vi "32路模拟量输入.vi"() -> ()   [LabVIEW 2010]
uses:
  全局量/全局_配置.vi
panel:
  in  "同步_1":i32
  in  "数组_反馈值":dbl[][](array[numeric])
  in  "第几个数据":i32
  in  "第几组数据":i32
  out "数组_AD幅值":sgl[](array[numeric])
  out "数组_DSP幅值":sgl[](array[numeric])
  in  "数组_设定值":dbl[][](array[numeric])
  in  "数组_选择":bool[](array[boolean])
  out "light_32":bool
  out "light_31":bool
  out "light_30":bool
  out "light_29":bool
  out "light_28":bool
  out "light_27":bool
  out "light_26":bool
  out "light_25":bool
  out "light_24":bool
  out "light_23":bool
  out "light_22":bool
  out "light_21":bool
  out "light_20":bool
  out "light_19":bool
  out "light_18":bool
  out "light_17":bool
  out "Analog_back":string[][](table) caption="表格"
  in  "A_32":bool
  in  "A_31":bool
  in  "A_30":bool
  in  "A_29":bool
  in  "A_28":bool
  in  "A_27":bool
  in  "A_26":bool
  in  "A_25":bool
  in  "A_24":bool
  in  "A_23":bool
  in  "A_22":bool
  in  "A_21":bool
  in  "A_20":bool
  in  "A_19":bool
  in  "A_18":bool
  in  "A_17":bool
  out "合格？":bool[][](array[boolean])
  out "测试结论":string
  out "light_16":bool
  out "light_15":bool
  out "light_14":bool
  out "light_13":bool
  out "light_12":bool
  out "light_11":bool
  out "light_10":bool
  out "light_9":bool
  out "light_8":bool
  out "light_7":bool
  out "light_6":bool
  out "light_5":bool
  out "light_4":bool
  out "light_3":bool
  out "light_2":bool
  out "light_1":bool
  out "退出？":bool
  in  "btn_反选":bool
  in  "btn_全选":bool
  in  "A_16":bool
  in  "A_15":bool
  in  "A_14":bool
  in  "A_13":bool
  in  "A_12":bool
  in  "A_11":bool
  in  "A_10":bool
  in  "A_9":bool
  in  "A_8":bool
  in  "A_7":bool
  in  "A_6":bool
  in  "A_5":bool
  in  "A_4":bool
  in  "A_3":bool
  in  "A_2":bool
  in  "A_1":bool
  in  "btn_取消":bool
  in  "btn_开始测试":bool
  in  "Analog_IN":string[][](table) caption="表格"
  out "Analog_WC":string[][](table) caption="表格"
  # "模拟量选择及输入值（V）"
  # "模拟量反馈值（V）"
  # "模拟量误差值（%）"
  # "测试结论："
  # "从0开始"
  # "从1开始,第0列没有使用"
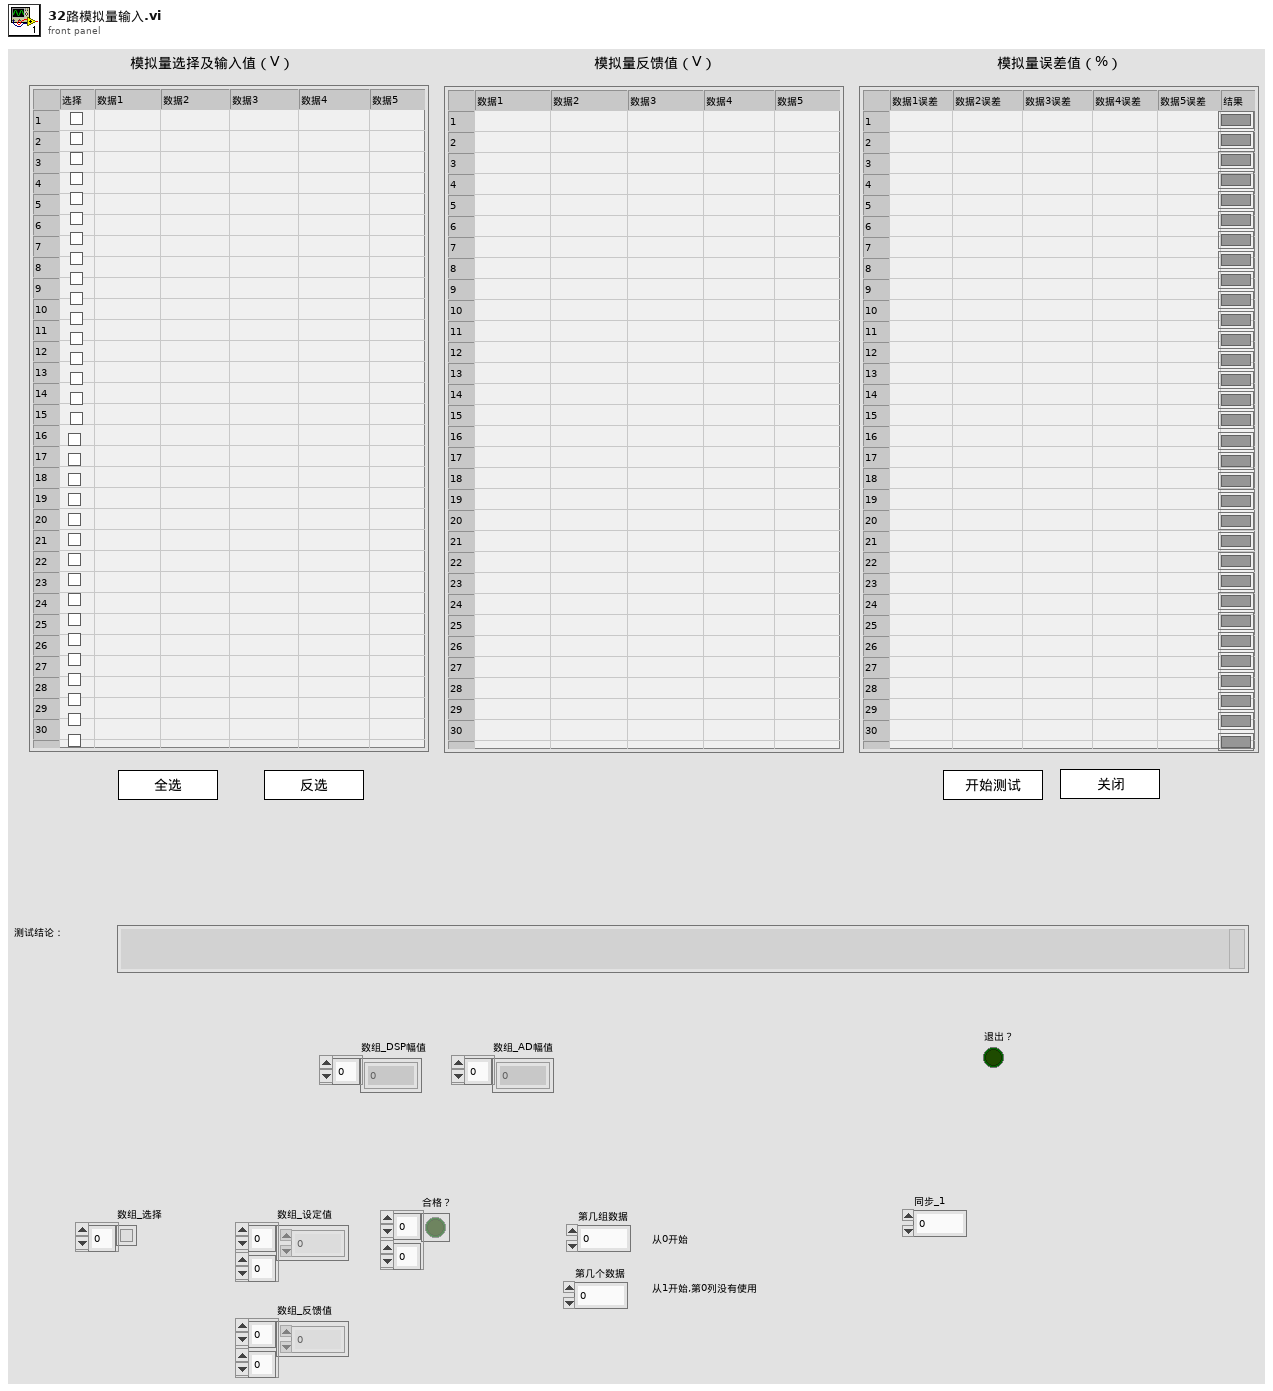
[diagram p1: front panel]
types:
  T1 = enum8{"Enabled", "Disabled", "Disabled and Grayed Out"}
  T2 = cluster{"数字量输入信号路数":u32, "数字量输出信号路数":u32, "DSP模拟量输入信号路数":u32, "DSP模拟量输入信号幅值":u32, "AD模拟量输入信号路数":u32, "AD模拟量输入信号幅值":u32, "RS232端口":u32, "RS232通信路数":u32, "RS232波特率":u32, "RS485端口":u32, "RS485通信路数":u32, "RS485波特率":u32, "CAN通信端口":string, "CAN波特率":u32, "以太网选择?":bool, "控制板IP":string, "以太网端口":u32}
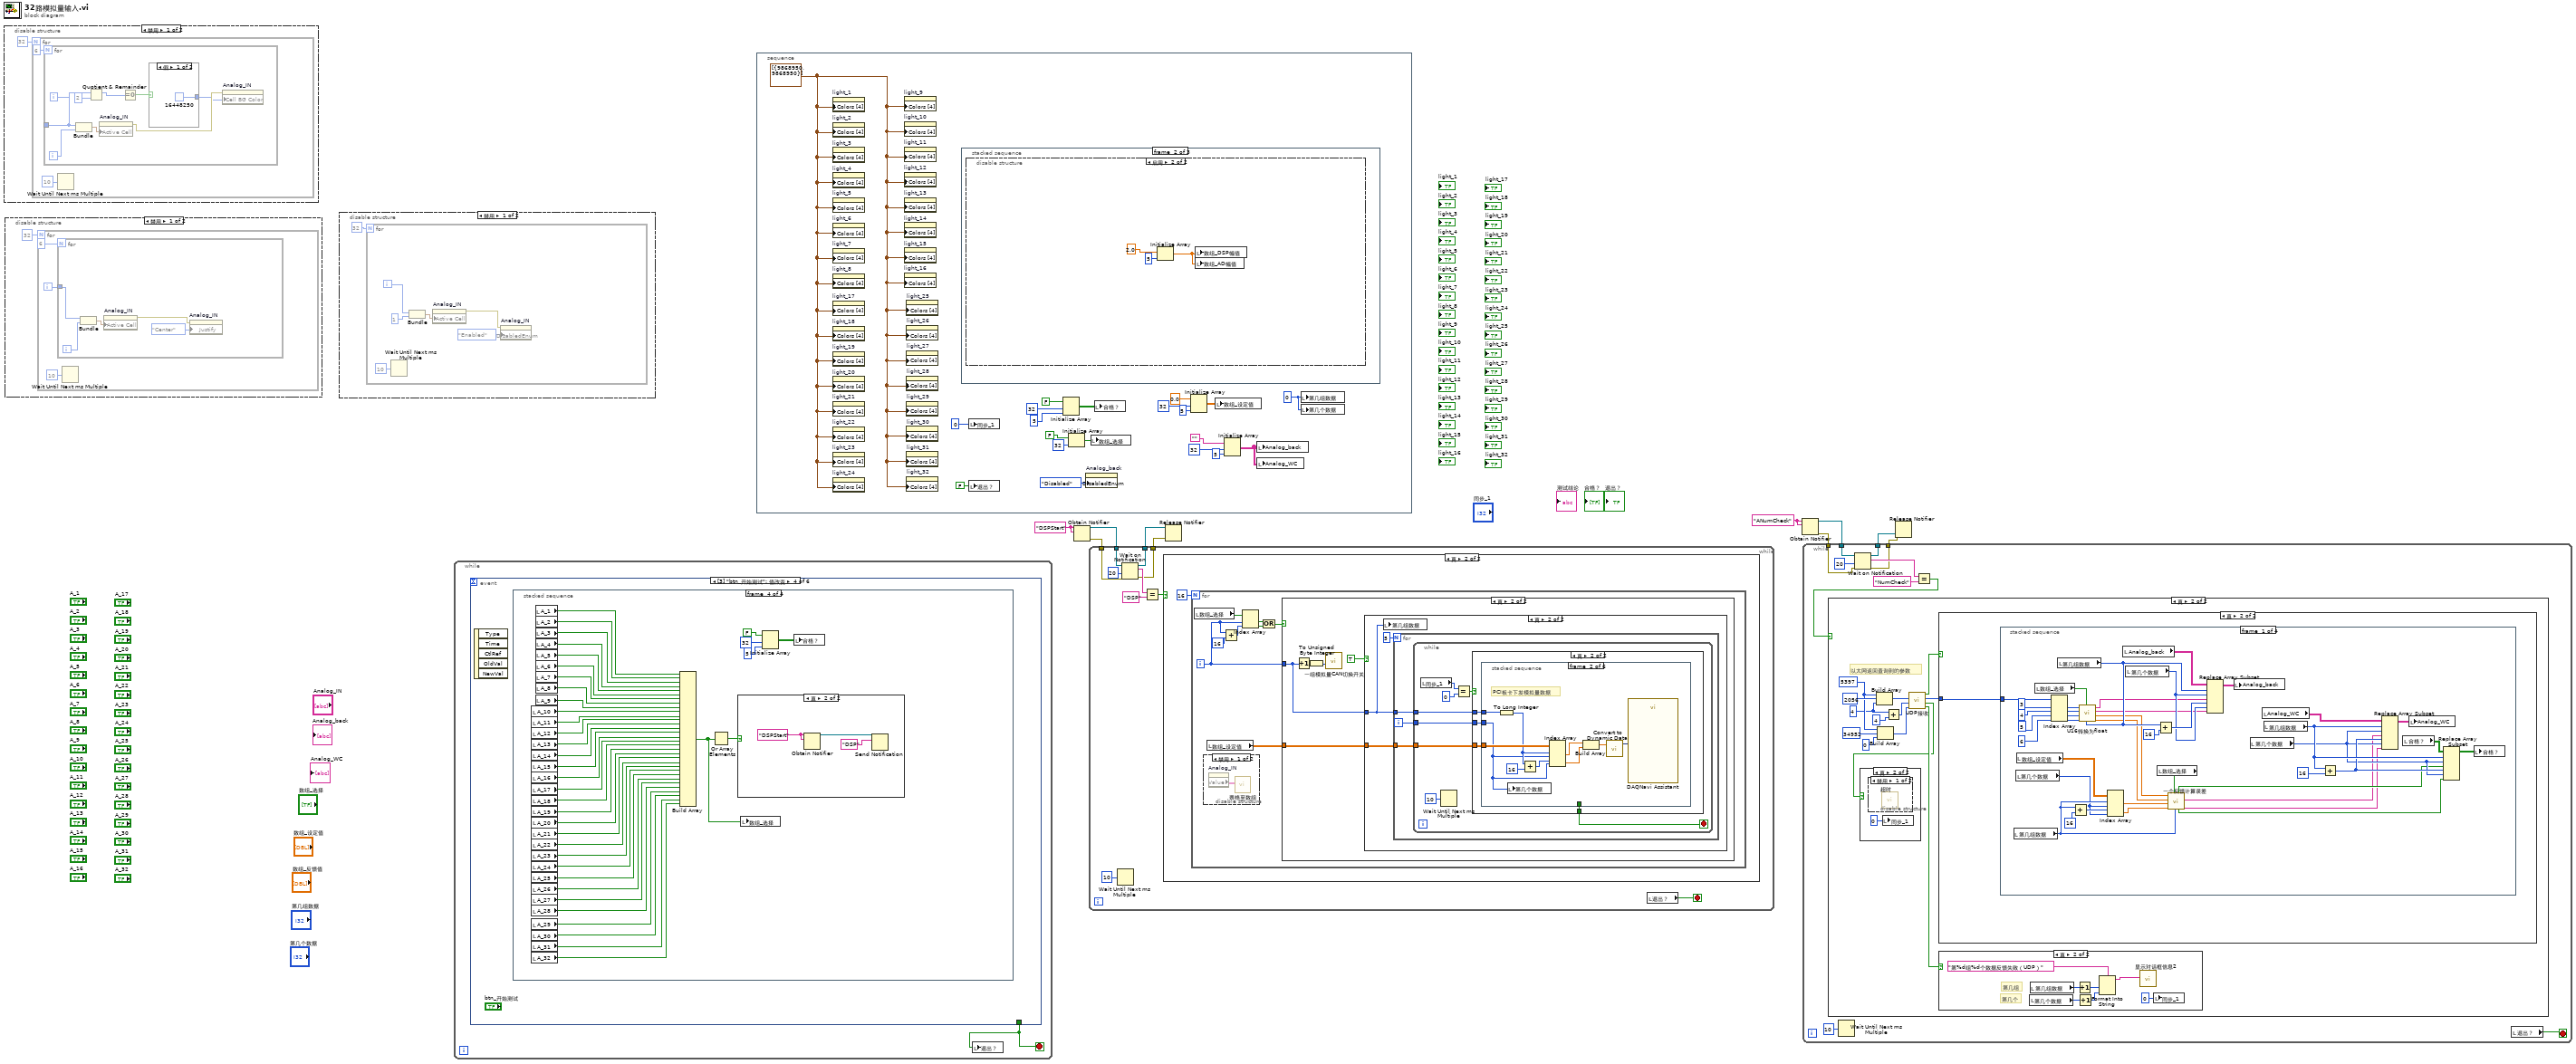
[diagram p0: block diagram]
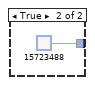
[diagram p2: hidden frame]
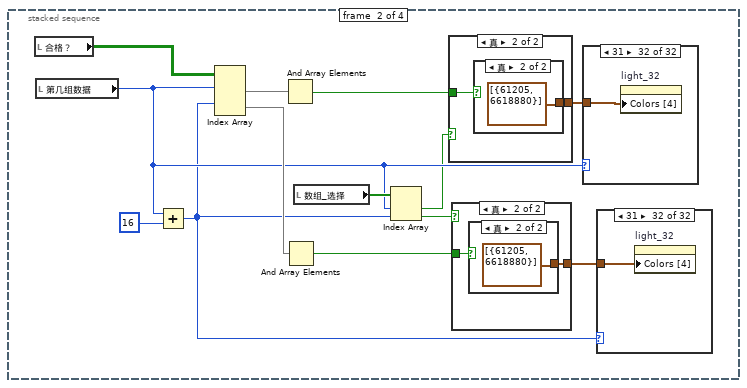
[diagram p9: hidden frame]
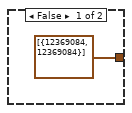
[diagram p10: hidden frame]
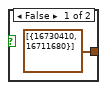
[diagram p11: hidden frame]
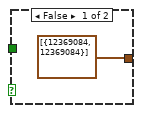
[diagram p12: hidden frame]
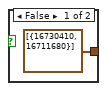
[diagram p13: hidden frame]
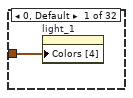
[diagram p14: hidden frame]
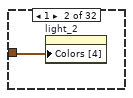
[diagram p15: hidden frame]
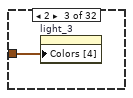
[diagram p16: hidden frame]
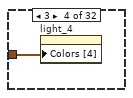
[diagram p17: hidden frame]
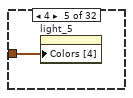
[diagram p18: hidden frame]
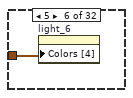
[diagram p19: hidden frame]
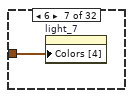
[diagram p20: hidden frame]
diagram:
  w5 = "ANumCheck" ("名称（未命名）")
  w8 = "DSPStart" ("名称（未命名）")
  n1 = disable-structure shown="禁用" {
    frame Disabled {
      n2 = for {
        N: 32 -> [_]
        i -> [w13]
        n3 = for {
          N: 6 -> [_]
          tunnel: w13 -> [w21]
          i -> [w15]
          n4 = Bundle(w21, w15) -> (w18:cluster{i32, i32})  [unwired: 1 in]
          n5 = Quotient & Remainder(x=w21, y=2) -> (x-y*floor(x/y)=w19:i32)  [unwired: 1 out]
          n6 = property on="Analog_IN" class="Tbl (严格)"("Active Cell"=w18) -> (error out=w17:errorcluster)  [unwired: 2 in, 1 out]
          n7 = Equal To 0?(x=w19) -> (x = 0?=w22:bool)
          n8 = case shown="假" w22 {
            tunnel: [u32 16448250 u32 15723488] -> w16
            frame False {
            }
            frame True {
            }
          }
          n9 = property on="Analog_IN" class="Tbl (严格)"(error in=w17, "Cell BG Color"=w16) -> ()  [unwired: 1 in, 2 out]
        }
        n10 = Wait Until Next ms Multiple(millisecond multiple=u32 10 ("毫秒倍数")) -> ()  [unwired: 1 out]
      }
    }
    frame Enabled {
    }
  }
  n11 = disable-structure shown="禁用" {
    frame Disabled {
      n12 = for {
        N: 32 -> [_]
        i -> [w26]
        n13 = for {
          N: 6 -> [_]
          tunnel: w26 -> [w29]
          i -> [w30]
          n14 = Bundle(w29, w30) -> (w33:cluster{i32, i32})  [unwired: 1 in]
          n15 = property on="Analog_IN" class="Tbl (严格)"("Active Cell"=w33) -> (error out=w31:errorcluster)  [unwired: 2 in, 1 out]
          n16 = property on="Analog_IN" class="Tbl (严格)"(error in=w31, "Justify"=enum16{"Left", "Center", "Right"}."Center" ("活动单元格:单元格对齐")) -> ()  [unwired: 1 in, 2 out]
        }
        n17 = Wait Until Next ms Multiple(millisecond multiple=u32 10 ("毫秒倍数")) -> ()  [unwired: 1 out]
      }
    }
    frame Enabled {
    }
  }
  n18 = disable-structure shown="禁用" {
    frame Disabled {
      n19 = for {
        N: 32 -> [_]
        i -> [w39]
        n20 = Wait Until Next ms Multiple(millisecond multiple=u32 10 ("毫秒倍数")) -> ()  [unwired: 1 out]
        n21 = Bundle(w39, 1) -> (w38:cluster{i32, i32})  [unwired: 1 in]
        n22 = property on="Analog_IN" class="Tbl (严格)"("Active Cell"=w38) -> (error out=w35:errorcluster)  [unwired: 2 in, 1 out]
        n23 = property on="Analog_IN" class="Tbl (严格)"(error in=w35, "DisabledEnum"=T1."Enabled" ("禁用")) -> ()  [unwired: 1 in, 2 out]
      }
    }
    frame Enabled {
    }
  }
  n24 = while {
    stop <- w41 stop-if-true
    n25 = event shown="[3] \"btn_开始测试\": 值改变" {
      selector: _ -> [_ _ _ _ _ _]
      dyn-events: _ -> [_ _ _ _ _ _]
      timeout: _ -> [_ _ _ _ _ _]
      tunnel: [_ TRUE TRUE _ _ _] -> w41
      event Timeout {
        n26 = event-data() -> ()  [unwired: 1 in, 2 out]
      }
      event Panel Close {
        n27 = event-data() -> ()  [unwired: 1 in, 3 out]
      }
      event "btn_取消": Value Change {
        n28 = event-data() -> ()  [unwired: 1 in, 5 out]
      }
      event "btn_开始测试": Value Change {
        n29 = event-data() -> ()  [unwired: 1 in, 5 out]
        n30 = stacked-sequence {
          frame #0 {
            w44 = 0 ("第几组数据")
            n31 = local read "Analog_IN"() -> (w51:string[][])
            n32 = Delete From Array(array=w51, length=1 ("长度"), index (col)=0 ("禁用的索引 (列)")) -> (array with subset deleted=w47:string[][])  [unwired: 1 in, 1 out]
            n33 = for {
              N: 32 -> [_]
              tunnel: w47 -> [w54] mode=indexing
              tunnel: [w53] -> w50 mode=indexing
              n34 = for {
                N: 5 -> [_]
                tunnel: w54 -> [w56] mode=indexing
                tunnel: [w55] -> w53 mode=indexing
                n35 = Fract/Exp String To Number(string=w56) -> (number=w55:dbl)  [unwired: 3 in, 1 out]
              }
            }
            n36 = local write "第几组数据"(w44) -> ()
            n37 = local write "第几个数据"(w44) -> ()
            n38 = local write "同步_1"(0 ("同步_2")) -> ()
            n39 = local write "数组_设定值"(w50) -> ()
          }
          frame #1 {
            n40 = local read "Analog_back"() -> (w59:string[][])
            n41 = local read "Analog_WC"() -> (w58:string[][])
            n42 = for {
              tunnel: w58 -> [w95] mode=indexing
              i -> [w94]
              n43 = for {
                tunnel: w95 -> [_] mode=indexing
                tunnel: w94 -> [w99]
                i -> [w98]
                n44 = local read "Analog_WC"() -> (w100:string[][])
                n45 = Replace Array Subset(array=w100, new element="", index (row)=w99, index (col)=w98) -> (w96:string[][])
                n46 = local write "Analog_WC"(w96) -> ()
              }
            }
            n47 = for {
              tunnel: w59 -> [w102] mode=indexing
              i -> [w101]
              n48 = for {
                tunnel: w102 -> [_] mode=indexing
                tunnel: w101 -> [w106]
                i -> [w105]
                n49 = local read "Analog_back"() -> (w107:string[][])
                n50 = Replace Array Subset(array=w107, new element="", index (row)=w106, index (col)=w105) -> (w103:string[][])
                n51 = local write "Analog_back"(w103) -> ()
              }
            }
            n52 = for {
              N: 32 -> [_]
              i -> [w61]
              n53 = case shown="31" w61 {
                tunnel: cluster{u32, u32}[] [{9868950, 9868950}] -> [w62 w63 w64 w65 w66 w67 w68 w69 w70 w71 w72 w73 w74 w75 w76 w77 w78 w79 w80 w81 w82 w83 w84 w85 w86 w87 w88 w89 w90 w91 w92 w93]
                frame 0, Default {
                  n54 = property on="light_1" class="Bool (严格)"("Colors [4]"=w62) -> ()  [unwired: 2 in, 2 out]
                }
                frame 1 {
                  n55 = property on="light_2" class="Bool (严格)"("Colors [4]"=w63) -> ()  [unwired: 2 in, 2 out]
                }
                frame 2 {
                  n56 = property on="light_3" class="Bool (严格)"("Colors [4]"=w64) -> ()  [unwired: 2 in, 2 out]
                }
                frame 3 {
                  n57 = property on="light_4" class="Bool (严格)"("Colors [4]"=w65) -> ()  [unwired: 2 in, 2 out]
                }
                frame 4 {
                  n58 = property on="light_5" class="Bool (严格)"("Colors [4]"=w66) -> ()  [unwired: 2 in, 2 out]
                }
                frame 5 {
                  n59 = property on="light_6" class="Bool (严格)"("Colors [4]"=w67) -> ()  [unwired: 2 in, 2 out]
                }
                frame 6 {
                  n60 = property on="light_7" class="Bool (严格)"("Colors [4]"=w68) -> ()  [unwired: 2 in, 2 out]
                }
                frame 7 {
                  n61 = property on="light_8" class="Bool (严格)"("Colors [4]"=w69) -> ()  [unwired: 2 in, 2 out]
                }
                frame 8 {
                  n62 = property on="light_9" class="Bool (严格)"("Colors [4]"=w70) -> ()  [unwired: 2 in, 2 out]
                }
                frame 9 {
                  n63 = property on="light_10" class="Bool (严格)"("Colors [4]"=w71) -> ()  [unwired: 2 in, 2 out]
                }
                frame 10 {
                  n64 = property on="light_11" class="Bool (严格)"("Colors [4]"=w72) -> ()  [unwired: 2 in, 2 out]
                }
                frame 11 {
                  n65 = property on="light_12" class="Bool (严格)"("Colors [4]"=w73) -> ()  [unwired: 2 in, 2 out]
                }
                frame 12 {
                  n66 = property on="light_13" class="Bool (严格)"("Colors [4]"=w74) -> ()  [unwired: 2 in, 2 out]
                }
                frame 13 {
                  n67 = property on="light_14" class="Bool (严格)"("Colors [4]"=w75) -> ()  [unwired: 2 in, 2 out]
                }
                frame 14 {
                  n68 = property on="light_15" class="Bool (严格)"("Colors [4]"=w76) -> ()  [unwired: 2 in, 2 out]
                }
                frame 15 {
                  n69 = property on="light_16" class="Bool (严格)"("Colors [4]"=w77) -> ()  [unwired: 2 in, 2 out]
                }
                frame 16 {
                  n70 = property on="light_17" class="Bool (严格)"("Colors [4]"=w78) -> ()  [unwired: 2 in, 2 out]
                }
                frame 17 {
                  n71 = property on="light_18" class="Bool (严格)"("Colors [4]"=w79) -> ()  [unwired: 2 in, 2 out]
                }
                frame 18 {
                  n72 = property on="light_19" class="Bool (严格)"("Colors [4]"=w80) -> ()  [unwired: 2 in, 2 out]
                }
                frame 19 {
                  n73 = property on="light_20" class="Bool (严格)"("Colors [4]"=w81) -> ()  [unwired: 2 in, 2 out]
                }
                frame 20 {
                  n74 = property on="light_21" class="Bool (严格)"("Colors [4]"=w82) -> ()  [unwired: 2 in, 2 out]
                }
                frame 21 {
                  n75 = property on="light_22" class="Bool (严格)"("Colors [4]"=w83) -> ()  [unwired: 2 in, 2 out]
                }
                frame 22 {
                  n76 = property on="light_23" class="Bool (严格)"("Colors [4]"=w84) -> ()  [unwired: 2 in, 2 out]
                }
                frame 23 {
                  n77 = property on="light_24" class="Bool (严格)"("Colors [4]"=w85) -> ()  [unwired: 2 in, 2 out]
                }
                frame 24 {
                  n78 = property on="light_25" class="Bool (严格)"("Colors [4]"=w86) -> ()  [unwired: 2 in, 2 out]
                }
                frame 25 {
                  n79 = property on="light_26" class="Bool (严格)"("Colors [4]"=w87) -> ()  [unwired: 2 in, 2 out]
                }
                frame 26 {
                  n80 = property on="light_27" class="Bool (严格)"("Colors [4]"=w88) -> ()  [unwired: 2 in, 2 out]
                }
                frame 27 {
                  n81 = property on="light_28" class="Bool (严格)"("Colors [4]"=w89) -> ()  [unwired: 2 in, 2 out]
                }
                frame 28 {
                  n82 = property on="light_29" class="Bool (严格)"("Colors [4]"=w90) -> ()  [unwired: 2 in, 2 out]
                }
                frame 29 {
                  n83 = property on="light_30" class="Bool (严格)"("Colors [4]"=w91) -> ()  [unwired: 2 in, 2 out]
                }
                frame 30 {
                  n84 = property on="light_31" class="Bool (严格)"("Colors [4]"=w92) -> ()  [unwired: 2 in, 2 out]
                }
                frame 31 {
                  n85 = property on="light_32" class="Bool (严格)"("Colors [4]"=w93) -> ()  [unwired: 2 in, 2 out]
                }
              }
            }
          }
          frame #2 {
            n86 = for {
              N: 32 -> [_]
              i -> [w110]
              n87 = disable-structure shown="禁用" {
                frame Disabled {
                  n88 = Wait Until Next ms Multiple(millisecond multiple=u32 10 ("毫秒倍数")) -> ()  [unwired: 1 out]
                }
                frame Enabled {
                }
              }
              n89 = for {
                N: 6 -> [_]
                tunnel: w110 -> [w118]
                i -> [w115]
                n90 = Bundle(w118, w115) -> (w114:cluster{i32, i32})  [unwired: 1 in]
                n91 = Quotient & Remainder(x=w118, y=2) -> (x-y*floor(x/y)=w116:i32)  [unwired: 1 out]
                n92 = property on="Analog_WC" class="Tbl (严格)"("Active Cell"=w114) -> (error out=w113:errorcluster)  [unwired: 2 in, 1 out]
                n93 = Equal To 0?(x=w116) -> (x = 0?=w119:bool)
                n94 = case shown="假" w119 {
                  tunnel: [u32 16448250 u32 15723488] -> w112
                  frame False {
                  }
                  frame True {
                  }
                }
                n95 = property on="Analog_WC" class="Tbl (严格)"(error in=w113, "Cell BG Color"=w112) -> ()  [unwired: 1 in, 2 out]
              }
            }
          }
          frame #3 {
            n96 = local read "A_10"() -> (w150:bool)
            n97 = local read "A_11"() -> (w149:bool)
            n98 = local read "A_12"() -> (w148:bool)
            n99 = local read "A_13"() -> (w147:bool)
            n100 = local read "A_14"() -> (w146:bool)
            n101 = local read "A_15"() -> (w145:bool)
            n102 = local read "A_16"() -> (w144:bool)
            n103 = local read "A_17"() -> (w143:bool)
            n104 = local read "A_18"() -> (w142:bool)
            n105 = local read "A_19"() -> (w141:bool)
            n106 = local read "A_20"() -> (w140:bool)
            n107 = local read "A_21"() -> (w139:bool)
            n108 = local read "A_22"() -> (w138:bool)
            n109 = local read "A_23"() -> (w137:bool)
            n110 = local read "A_24"() -> (w136:bool)
            n111 = local read "A_25"() -> (w135:bool)
            n112 = local read "A_26"() -> (w134:bool)
            n113 = local read "A_27"() -> (w133:bool)
            n114 = local read "A_28"() -> (w132:bool)
            n115 = local read "A_29"() -> (w131:bool)
            n116 = local read "A_30"() -> (w130:bool)
            n117 = local read "A_31"() -> (w129:bool)
            n118 = local read "A_32"() -> (w128:bool)
            n119 = local read "A_1"() -> (w159:bool)
            n120 = local read "A_2"() -> (w158:bool)
            n121 = local read "A_3"() -> (w157:bool)
            n122 = local read "A_4"() -> (w156:bool)
            n123 = local read "A_5"() -> (w155:bool)
            n124 = local read "A_6"() -> (w154:bool)
            n125 = local read "A_7"() -> (w153:bool)
            n126 = local read "A_8"() -> (w152:bool)
            n127 = local read "A_9"() -> (w151:bool)
            n128 = Build Array(w159, w158, w157, w156, w155, w154, w153, w152, w151, w150, w149, w148, w147, w146, w145, w144, w143, w142, w141, w140, w139, w138, w137, w136, w135, w134, w133, w132, w131, w130, w129, w128) -> (w122:bool[])
            n129 = Or Array Elements(Boolean array=w122) -> (logical OR=w127:bool)
            n130 = case shown="真" w127 {
              frame False {
                n131 = call "显示对话框信息"() -> ()  [unwired: 10 in, 2 out]
              }
              frame True {
                w161 = "DSPStart" ("名称（未命名）")
                n132 = Obtain Notifier(name (unnamed)=w161, notification data type=w161) -> (notifier out=w160:refnum<notifier>)  [unwired: 2 in, 2 out]
                n133 = Send Notification(notification="DSP" ("通知"), notifier=w160) -> ()  [unwired: 1 in, 2 out]
              }
            }
            n134 = local write "数组_选择"(w122) -> ()
            n135 = Initialize Array(FALSE, 32 ("维数大小"), 5 ("维数大小")) -> (w123:bool[][])
            n136 = local write "合格？"(w123) -> ()
          }
        }
      }
      event "btn_全选": Value Change {
        w163 = TRUE ("单选_AD_1")
        n137 = event-data() -> ()  [unwired: 1 in, 5 out]
        n138 = local write "A_1"(w163) -> ()
        n139 = local write "A_2"(w163) -> ()
        n140 = local write "A_3"(w163) -> ()
        n141 = local write "A_4"(w163) -> ()
        n142 = local write "A_5"(w163) -> ()
        n143 = local write "A_6"(w163) -> ()
        n144 = local write "A_7"(w163) -> ()
        n145 = local write "A_8"(w163) -> ()
        n146 = local write "A_9"(w163) -> ()
        n147 = local write "A_10"(w163) -> ()
        n148 = local write "A_11"(w163) -> ()
        n149 = local write "A_12"(w163) -> ()
        n150 = local write "A_13"(w163) -> ()
        n151 = local write "A_14"(w163) -> ()
        n152 = local write "A_15"(w163) -> ()
        n153 = local write "A_16"(w163) -> ()
        n154 = local write "A_17"(w163) -> ()
        n155 = local write "A_18"(w163) -> ()
        n156 = local write "A_19"(w163) -> ()
        n157 = local write "A_20"(w163) -> ()
        n158 = local write "A_21"(w163) -> ()
        n159 = local write "A_22"(w163) -> ()
        n160 = local write "A_23"(w163) -> ()
        n161 = local write "A_24"(w163) -> ()
        n162 = local write "A_25"(w163) -> ()
        n163 = local write "A_26"(w163) -> ()
        n164 = local write "A_27"(w163) -> ()
        n165 = local write "A_28"(w163) -> ()
        n166 = local write "A_29"(w163) -> ()
        n167 = local write "A_30"(w163) -> ()
        n168 = local write "A_31"(w163) -> ()
        n169 = local write "A_32"(w163) -> ()
      }
      event "btn_反选": Value Change {
        n170 = event-data() -> ()  [unwired: 1 in, 5 out]
        n171 = local read "A_17"() -> (w195:bool)
        n172 = local read "A_18"() -> (w193:bool)
        n173 = local read "A_19"() -> (w191:bool)
        n174 = local read "A_20"() -> (w189:bool)
        n175 = local read "A_21"() -> (w187:bool)
        n176 = local read "A_22"() -> (w185:bool)
        n177 = local read "A_23"() -> (w183:bool)
        n178 = local read "A_24"() -> (w181:bool)
        n179 = local read "A_25"() -> (w179:bool)
        n180 = local read "A_26"() -> (w177:bool)
        n181 = local read "A_27"() -> (w175:bool)
        n182 = local read "A_28"() -> (w173:bool)
        n183 = local read "A_29"() -> (w171:bool)
        n184 = local read "A_30"() -> (w169:bool)
        n185 = local read "A_31"() -> (w167:bool)
        n186 = local read "A_32"() -> (w165:bool)
        n187 = local read "A_1"() -> (w227:bool)
        n188 = local read "A_2"() -> (w225:bool)
        n189 = local read "A_3"() -> (w224:bool)
        n190 = local read "A_4"() -> (w223:bool)
        n191 = local read "A_5"() -> (w222:bool)
        n192 = local read "A_6"() -> (w221:bool)
        n193 = local read "A_7"() -> (w220:bool)
        n194 = local read "A_8"() -> (w219:bool)
        n195 = local read "A_9"() -> (w218:bool)
        n196 = local read "A_10"() -> (w217:bool)
        n197 = local read "A_11"() -> (w216:bool)
        n198 = local read "A_12"() -> (w215:bool)
        n199 = local read "A_13"() -> (w214:bool)
        n200 = local read "A_14"() -> (w213:bool)
        n201 = local read "A_15"() -> (w212:bool)
        n202 = local read "A_16"() -> (w211:bool)
        n203 = Not(x=w227) -> (.not. x?=w226:bool)
        n204 = Not(x=w225) -> (.not. x?=w196:bool)
        n205 = Not(x=w224) -> (.not. x?=w197:bool)
        n206 = Not(x=w223) -> (.not. x?=w198:bool)
        n207 = Not(x=w222) -> (.not. x?=w199:bool)
        n208 = Not(x=w221) -> (.not. x?=w200:bool)
        n209 = Not(x=w220) -> (.not. x?=w201:bool)
        n210 = Not(x=w219) -> (.not. x?=w202:bool)
        n211 = Not(x=w218) -> (.not. x?=w203:bool)
        n212 = Not(x=w217) -> (.not. x?=w204:bool)
        n213 = Not(x=w216) -> (.not. x?=w205:bool)
        n214 = Not(x=w215) -> (.not. x?=w206:bool)
        n215 = Not(x=w214) -> (.not. x?=w207:bool)
        n216 = Not(x=w213) -> (.not. x?=w208:bool)
        n217 = Not(x=w212) -> (.not. x?=w209:bool)
        n218 = Not(x=w211) -> (.not. x?=w210:bool)
        n219 = Not(x=w195) -> (.not. x?=w194:bool)
        n220 = Not(x=w193) -> (.not. x?=w192:bool)
        n221 = Not(x=w191) -> (.not. x?=w190:bool)
        n222 = Not(x=w189) -> (.not. x?=w188:bool)
        n223 = Not(x=w187) -> (.not. x?=w186:bool)
        n224 = Not(x=w185) -> (.not. x?=w184:bool)
        n225 = Not(x=w183) -> (.not. x?=w182:bool)
        n226 = Not(x=w181) -> (.not. x?=w180:bool)
        n227 = Not(x=w179) -> (.not. x?=w178:bool)
        n228 = Not(x=w177) -> (.not. x?=w176:bool)
        n229 = Not(x=w175) -> (.not. x?=w174:bool)
        n230 = Not(x=w173) -> (.not. x?=w172:bool)
        n231 = Not(x=w171) -> (.not. x?=w170:bool)
        n232 = Not(x=w169) -> (.not. x?=w168:bool)
        n233 = Not(x=w167) -> (.not. x?=w166:bool)
        n234 = Not(x=w165) -> (.not. x?=w164:bool)
        n235 = local write "A_1"(w226) -> ()
        n236 = local write "A_2"(w196) -> ()
        n237 = local write "A_3"(w197) -> ()
        n238 = local write "A_4"(w198) -> ()
        n239 = local write "A_5"(w199) -> ()
        n240 = local write "A_6"(w200) -> ()
        n241 = local write "A_7"(w201) -> ()
        n242 = local write "A_8"(w202) -> ()
        n243 = local write "A_9"(w203) -> ()
        n244 = local write "A_10"(w204) -> ()
        n245 = local write "A_11"(w205) -> ()
        n246 = local write "A_12"(w206) -> ()
        n247 = local write "A_13"(w207) -> ()
        n248 = local write "A_14"(w208) -> ()
        n249 = local write "A_15"(w209) -> ()
        n250 = local write "A_16"(w210) -> ()
        n251 = local write "A_17"(w194) -> ()
        n252 = local write "A_18"(w192) -> ()
        n253 = local write "A_19"(w190) -> ()
        n254 = local write "A_20"(w188) -> ()
        n255 = local write "A_21"(w186) -> ()
        n256 = local write "A_22"(w184) -> ()
        n257 = local write "A_23"(w182) -> ()
        n258 = local write "A_24"(w180) -> ()
        n259 = local write "A_25"(w178) -> ()
        n260 = local write "A_26"(w176) -> ()
        n261 = local write "A_27"(w174) -> ()
        n262 = local write "A_28"(w172) -> ()
        n263 = local write "A_29"(w170) -> ()
        n264 = local write "A_30"(w168) -> ()
        n265 = local write "A_31"(w166) -> ()
        n266 = local write "A_32"(w164) -> ()
      }
    }
    n267 = local write "退出？"(w41) -> ()
  }
  n268 = stacked-sequence {
    frame #0 {
      w228 = 0 ("第几组数据")
      w243 = cluster{u32, u32}[] [{9868950, 9868950}]
      n269 = property on="light_1" class="Bool (严格)"("Colors [4]"=w243) -> ()  [unwired: 2 in, 2 out]
      n270 = property on="light_2" class="Bool (严格)"("Colors [4]"=w243) -> ()  [unwired: 2 in, 2 out]
      n271 = property on="light_3" class="Bool (严格)"("Colors [4]"=w243) -> ()  [unwired: 2 in, 2 out]
      n272 = property on="light_4" class="Bool (严格)"("Colors [4]"=w243) -> ()  [unwired: 2 in, 2 out]
      n273 = property on="light_5" class="Bool (严格)"("Colors [4]"=w243) -> ()  [unwired: 2 in, 2 out]
      n274 = property on="light_6" class="Bool (严格)"("Colors [4]"=w243) -> ()  [unwired: 2 in, 2 out]
      n275 = property on="light_7" class="Bool (严格)"("Colors [4]"=w243) -> ()  [unwired: 2 in, 2 out]
      n276 = property on="light_8" class="Bool (严格)"("Colors [4]"=w243) -> ()  [unwired: 2 in, 2 out]
      n277 = property on="light_17" class="Bool (严格)"("Colors [4]"=w243) -> ()  [unwired: 2 in, 2 out]
      n278 = property on="light_18" class="Bool (严格)"("Colors [4]"=w243) -> ()  [unwired: 2 in, 2 out]
      n279 = property on="light_19" class="Bool (严格)"("Colors [4]"=w243) -> ()  [unwired: 2 in, 2 out]
      n280 = property on="light_20" class="Bool (严格)"("Colors [4]"=w243) -> ()  [unwired: 2 in, 2 out]
      n281 = property on="light_21" class="Bool (严格)"("Colors [4]"=w243) -> ()  [unwired: 2 in, 2 out]
      n282 = property on="light_22" class="Bool (严格)"("Colors [4]"=w243) -> ()  [unwired: 2 in, 2 out]
      n283 = property on="light_23" class="Bool (严格)"("Colors [4]"=w243) -> ()  [unwired: 2 in, 2 out]
      n284 = property on="light_24" class="Bool (严格)"("Colors [4]"=w243) -> ()  [unwired: 2 in, 2 out]
      n285 = property on="light_9" class="Bool (严格)"("Colors [4]"=w243) -> ()  [unwired: 2 in, 2 out]
      n286 = property on="light_10" class="Bool (严格)"("Colors [4]"=w243) -> ()  [unwired: 2 in, 2 out]
      n287 = property on="light_11" class="Bool (严格)"("Colors [4]"=w243) -> ()  [unwired: 2 in, 2 out]
      n288 = property on="light_12" class="Bool (严格)"("Colors [4]"=w243) -> ()  [unwired: 2 in, 2 out]
      n289 = property on="light_13" class="Bool (严格)"("Colors [4]"=w243) -> ()  [unwired: 2 in, 2 out]
      n290 = property on="light_14" class="Bool (严格)"("Colors [4]"=w243) -> ()  [unwired: 2 in, 2 out]
      n291 = property on="light_15" class="Bool (严格)"("Colors [4]"=w243) -> ()  [unwired: 2 in, 2 out]
      n292 = property on="light_16" class="Bool (严格)"("Colors [4]"=w243) -> ()  [unwired: 2 in, 2 out]
      n293 = property on="light_25" class="Bool (严格)"("Colors [4]"=w243) -> ()  [unwired: 2 in, 2 out]
      n294 = property on="light_26" class="Bool (严格)"("Colors [4]"=w243) -> ()  [unwired: 2 in, 2 out]
      n295 = property on="light_27" class="Bool (严格)"("Colors [4]"=w243) -> ()  [unwired: 2 in, 2 out]
      n296 = property on="light_28" class="Bool (严格)"("Colors [4]"=w243) -> ()  [unwired: 2 in, 2 out]
      n297 = property on="light_29" class="Bool (严格)"("Colors [4]"=w243) -> ()  [unwired: 2 in, 2 out]
      n298 = property on="light_30" class="Bool (严格)"("Colors [4]"=w243) -> ()  [unwired: 2 in, 2 out]
      n299 = property on="light_31" class="Bool (严格)"("Colors [4]"=w243) -> ()  [unwired: 2 in, 2 out]
      n300 = property on="light_32" class="Bool (严格)"("Colors [4]"=w243) -> ()  [unwired: 2 in, 2 out]
      n301 = stacked-sequence {
        frame #0 {
          n302 = Initialize Array("", 32 ("维数大小"), 6 ("维数大小")) -> (w248:string[][])
          n303 = local write "Analog_IN"(w248) -> ()
        }
        frame #1 {
          n304 = disable-structure shown="启用" {
            frame Disabled {
              n305 = global read "全局_配置.vi" "BoardConfig"() -> (w256:T2)
              n306 = Unbundle By Name(w256) -> ("DSP模拟量输入信号幅值"=w255:u32, "AD模拟量输入信号幅值"=w254:u32)
              n307 = case shown="2" w254 {
                tunnel: [sgl 3.0 sgl 5.0 sgl 12.0] -> w252
                frame 0, Default {
                }
                frame 1 {
                }
                frame 2 {
                }
              }
              n308 = case shown="0, 默认" w255 {
                tunnel: [sgl 3.0 sgl 5.0 sgl 12.0] -> w253
                frame 0, Default {
                }
                frame 1 {
                }
                frame 2 {
                }
              }
              n309 = for {
                N: 5 -> [_]
                tunnel: w253 -> [w278]
                tunnel: w252 -> [w269]
                tunnel: [w267] -> w258 mode=indexing
                tunnel: [w266] -> w257 mode=indexing
                i -> [w281]
                n310 = Multiply(x=sgl 2.0, y=w278) -> (x*y=w276:sgl)
                n311 = Multiply(x=sgl 2.0, y=w269) -> (x*y=w273:sgl)
                n312 = case shown="4" w281 {
                  tunnel: [sgl 0.05 sgl 0.5 sgl 0.75 sgl 0.95 sgl 0.25] -> w268
                  frame 0, Default {
                  }
                  frame 2 {
                  }
                  frame 3 {
                  }
                  frame 4 {
                  }
                  frame 1 {
                  }
                }
                n313 = Multiply(x=w278, y=sgl -1.0) -> (x*y=w279:sgl)
                n314 = Multiply(x=w269, y=sgl -1.0) -> (x*y=w271:sgl)
                n315 = Multiply(x=w268, y=w276) -> (x*y=w275:sgl)
                n316 = Multiply(x=w268, y=w273) -> (x*y=w274:sgl)
                n317 = Add(x=w275, y=w279) -> (x+y=w267:sgl)
                n318 = Add(x=w274, y=w271) -> (x+y=w266:sgl)
              }
              "数组_DSP幅值" <- w258
              "数组_AD幅值" <- w257
            }
            frame Enabled {
              n319 = Initialize Array(sgl 2.0, 5 ("维数大小")) -> (w289:sgl[])
              n320 = local write "数组_DSP幅值"(w289) -> ()
              n321 = local write "数组_AD幅值"(w289) -> ()
            }
          }
        }
        frame #2 {
          n322 = stacked-sequence {
            frame #0 {
              n323 = for {
                N: 16 -> [_]
                i -> [w291]
                n324 = local read "数组_DSP幅值"() -> (w292:sgl[])
                n325 = for {
                  N: 5 -> [_]
                  tunnel: w292 -> [w299] mode=indexing
                  tunnel: w291 -> [w298]
                  i -> [w296]
                  n326 = local read "Analog_IN"() -> (w302:string[][])
                  n327 = Number To Fractional String(number=w299, precision (6)=i16 2 ("精度(6)")) -> (F-format string=w297:string)  [unwired: 2 in]
                  n328 = Increment(x=w296) -> (x+1=w295:i32)
                  n329 = Replace Array Subset(array=w302, new element=w297, index (row)=w298, index (col)=w295) -> (w301:string[][])
                  n330 = local write "Analog_IN"(w301) -> ()
                  n331 = Wait Until Next ms Multiple(millisecond multiple=u32 2 ("毫秒倍数")) -> ()  [unwired: 1 out]
                }
              }
            }
            frame #1 {
              n332 = for {
                N: 16 -> [_]
                i -> [w305]
                n333 = local read "数组_AD幅值"() -> (w304:sgl[])
                n334 = for {
                  N: 5 -> [_]
                  tunnel: w304 -> [w314] mode=indexing
                  tunnel: w305 -> [w309]
                  i -> [w312]
                  n335 = Add(x=w309, y=16) -> (x+y=w307:i32)
                  n336 = local read "Analog_IN"() -> (w317:string[][])
                  n337 = Number To Fractional String(number=w314, precision (6)=i16 2 ("精度(6)")) -> (F-format string=w313:string)  [unwired: 2 in]
                  n338 = Increment(x=w312) -> (x+1=w311:i32)
                  n339 = Replace Array Subset(array=w317, new element=w313, index (row)=w307, index (col)=w311) -> (w316:string[][])
                  n340 = local write "Analog_IN"(w316) -> ()
                  n341 = Wait Until Next ms Multiple(millisecond multiple=u32 2 ("毫秒倍数")) -> ()  [unwired: 1 out]
                }
              }
            }
          }
        }
      }
      n342 = local write "同步_1"(0 ("同步_2")) -> ()
      n343 = local write "退出？"(FALSE ("退出？")) -> ()
      n344 = Initialize Array(FALSE, 32 ("维数大小"), 5 ("维数大小")) -> (w244:bool[][])
      n345 = Initialize Array(FALSE, 32 ("维数大小")) -> (w232:bool[])
      n346 = property on="Analog_back" class="Tbl (严格)"("DisabledEnum"=T1."Disabled" ("禁用")) -> ()  [unwired: 2 in, 2 out]
      n347 = local write "数组_选择"(w232) -> ()
      n348 = local write "合格？"(w244) -> ()
      n349 = Initialize Array(0.0, 32 ("维数大小"), 5 ("维数大小")) -> (w235:dbl[][])
      n350 = local write "数组_设定值"(w235) -> ()
      n351 = Initialize Array("", 32 ("维数大小"), 5 ("维数大小")) -> (w239:string[][])
      n352 = local write "Analog_back"(w239) -> ()
      n353 = local write "Analog_WC"(w239) -> ()
      n354 = local write "第几组数据"(w228) -> ()
      n355 = local write "第几个数据"(w228) -> ()
    }
  }
  n356 = Obtain Notifier(name (unnamed)=w8, notification data type=w8) -> (notifier out=w10:refnum<notifier>, error out=w9:errorcluster)  [unwired: 2 in, 1 out]
  n357 = while {
    tunnel: w10 -> [w321]
    tunnel: w9 -> [w320]
    tunnel: [w319] -> w7
    tunnel: [w318] -> w6
    stop <- w323 stop-if-true
    n358 = Wait Until Next ms Multiple(millisecond multiple=u32 10 ("毫秒倍数")) -> ()  [unwired: 1 out]
    n359 = Wait on Notification(notifier=w321, timeout in ms (-1)=20 ("超时毫秒(-1)"), error in (no error)=w320) -> (notifier out=w319:refnum<notifier>, notification=w327:string, error out=w318:errorcluster)  [unwired: 1 in, 1 out]
    n360 = Equal?(x=w327, y="DSP" ("通知")) -> (x = y?=w324:bool)
    n361 = case shown="真" w324 {
      frame False {
      }
      frame True {
        n362 = for {
          N: 16 -> [_]
          i -> [w332]
          n363 = local read "数组_选择"() -> (w335:bool[])
          n364 = disable-structure shown="禁用" {
            frame Disabled {
              n365 = property on="Analog_IN" class="Tbl (严格)"() -> ("Value"=w337:string[][])  [unwired: 2 in, 2 out]
              n366 = call "表格至数组.vi"("表格控件"=w337) -> ()  [unwired: 10 in, 1 out]
            }
            frame Enabled {
            }
          }
          n367 = local read "数组_设定值"() -> (w336:dbl[][])
          n368 = Add(x=w332, y=16) -> (x+y=w333:i32)
          n369 = Index Array(array=w335, index #1=w332, index #2=w333) -> (element #1=w330:bool, element #2=w329:bool)
          n370 = Or(x=w330, y=w329) -> (x .or. y?=w334:bool)
          n371 = case shown="真" w334 {
            tunnel: w332 -> [_ w338]
            tunnel: w336 -> [_ w340]
            frame False {
            }
            frame True {
              n372 = Increment(x=w338) -> (x+1=w341:i32)
              n373 = To Unsigned Byte Integer(number=w341) -> (unsigned 8bit integer=w342:u8)
              n374 = call "一组模拟量CAN切换开关.vi"("第几组数据"=w342) -> ()  [unwired: 10 in, 1 out]
              n375 = case shown="真" TRUE {
                tunnel: w338 -> [_ w343]
                tunnel: w340 -> [_ w344]
                frame False {
                }
                frame True {
                  n376 = local write "第几组数据"(w343) -> ()
                  n377 = for {
                    N: 5 -> [_]
                    tunnel: w343 -> [w348]
                    tunnel: w344 -> [w347]
                    i -> [w346]
                    n378 = while {
                      tunnel: w348 -> [w356]
                      tunnel: w347 -> [w355]
                      tunnel: w346 -> [w354]
                      stop <- w351 stop-if-true
                      n379 = local read "同步_1"() -> (w352:i32)
                      n380 = Wait Until Next ms Multiple(millisecond multiple=u32 10 ("毫秒倍数")) -> ()  [unwired: 1 out]
                      n381 = Equal?(x=w352, y=0) -> (x = y?=w353:bool)
                      n382 = case shown="真" w353 {
                        tunnel: w356 -> [_ w361]
                        tunnel: w355 -> [_ w360]
                        tunnel: w354 -> [_ w359]
                        tunnel: [FALSE w358] -> w351
                        frame False {
                        }
                        frame True {
                          n383 = stacked-sequence {
                            tunnel: w361 -> [_ w367 _ _ w385 _]
                            tunnel: w360 -> [_ w370 _ _ _ _]
                            tunnel: w359 -> [_ w363 _ _ _ _]
                            tunnel: [_ _ _ _ _ w386] -> w358
                            frame #0 {
                              n384 = Wait (ms)(milliseconds to wait=u32 100) -> ()  [unwired: 1 out]
                            }
                            frame #1 {
                              # "PCI板卡下发模拟量数据"
                              n385 = To Long Integer(number=w367) -> (32bit integer=w366:i32)
                              n386 = local write "第几个数据"(w363) -> ()
                              n387 = Add(x=w366, y=16) -> (x+y=w368:i32)
                              n388 = Index Array(array=w370, index (row) #1=w366, index (col) #1=w363, index (row) #2=w368, index (col) #2=w363) -> (element #1=w365:dbl, element #2=w364:dbl)
                              n389 = Build Array(w365, w364) -> (w371:dbl[])
                              n390 = call "Convert to Dynamic Data"("Array"=w371) -> ("Dynamic Data Type"=w372:dynamicdata)  [unwired: 3 out]
                              n391 = call "DAQNavi Assistant"("data in(DDT)"=w372) -> ()  [unwired: 2 in, 17 out]
                            }
                            frame #2 {
                              w375 = "ANumCheck" ("名称（未命名）")
                              n392 = Obtain Notifier(name (unnamed)=w375, notification data type=w375) -> (notifier out=w374:refnum<notifier>)  [unwired: 2 in, 2 out]
                              n393 = local write "同步_1"(1 ("同步_1")) -> ()
                              n394 = Send Notification(notification="NumCheck" ("通知"), notifier=w374) -> ()  [unwired: 1 in, 2 out]
                            }
                            frame #3 {
                              n395 = Wait (ms)(milliseconds to wait=u32 150) -> ()  [unwired: 1 out]
                            }
                            frame #4 {
                              # "待定"
                              # "待定"
                              # "待定"
                              # "以太网发送读取参数命令"
                              n396 = To Unsigned Word Integer(number=w385) -> (unsigned 16bit integer=w381:u16)
                              n397 = Add(x=w381, y=u16 16) -> (x+y=w382:u16)
                              n398 = Build Array(w381, w382) -> (w384:u16[])
                              n399 = call "UDP发送.vi"("发送数据"=w384, "数据区字长"=u16 2, "报文类型"=u16 2056, "发送方标识"=u16 5397) -> ()  [unwired: 6 in, 1 out]
                            }
                            frame #5 {
                              n400 = local read "同步_1"() -> (w388:i32)
                              n401 = Equal?(x=w388, y=1) -> (x = y?=w386:bool)
                            }
                          }
                        }
                      }
                    }
                  }
                }
              }
            }
          }
        }
      }
    }
    n402 = local read "退出？"() -> (w323:bool)
  }
  n403 = Release Notifier(notifier=w7, error in (no error)=w6) -> ()  [unwired: 1 in, 3 out]
  n404 = Obtain Notifier(name (unnamed)=w5, notification data type=w5) -> (notifier out=w4:refnum<notifier>, error out=w3:errorcluster)  [unwired: 2 in, 1 out]
  n405 = while {
    tunnel: w4 -> [w393]
    tunnel: w3 -> [w392]
    tunnel: [w391] -> w2
    tunnel: [w390] -> w1
    stop <- w389 stop-if-true
    n406 = Wait Until Next ms Multiple(millisecond multiple=u32 10 ("毫秒倍数")) -> ()  [unwired: 1 out]
    n407 = Wait on Notification(notifier=w393, timeout in ms (-1)=20 ("超时毫秒(-1)"), error in (no error)=w392) -> (notifier out=w391:refnum<notifier>, notification=w396:string, error out=w390:errorcluster)  [unwired: 1 in, 1 out]
    n408 = Equal?(x=w396, y="NumCheck" ("通知")) -> (x = y?=w394:bool)
    n409 = case shown="真" w394 {
      frame False {
      }
      frame True {
        w401 = u16 4
        w410 = u16 5397
        # "以太网返回查询到的参数"
        n410 = Build Array(w410, u16 2056, w401) -> (w407:u16[])
        n411 = Build Array(w410, u16 34952, u16 0 ("元素")) -> (w406:u16[])
        n412 = Add(x=w401, y=u16 4) -> (x+y=w399:u16)
        n413 = call "UDP接收.vi"("匹配帧信息_异常"=w406, "长度"=w399, "匹配帧信息_正常"=w407) -> ("异常_找到?"=w403:bool, "接收超时?"=w402:bool, "接收的一帧数据"=w404:u16[], "正常_找到?"=w405:bool)  [unwired: 5 in]
        n414 = case shown="真" w402 {
          frame False {
          }
          frame True {
            n415 = disable-structure shown="禁用" {
              frame Disabled {
                n416 = call "超时"() -> ()  [unwired: 10 in, 2 out]
              }
              frame Enabled {
              }
            }
            n417 = local write "同步_1"(0 ("同步_1")) -> ()
          }
        }
        n418 = case shown="真" w405 {
          tunnel: w404 -> [_ w420]
          frame False {
          }
          frame True {
            n419 = stacked-sequence {
              tunnel: w420 -> [w460 _ _ _]
              frame #0 {
                n420 = local read "第几组数据"() -> (w428:i32)
                n421 = local read "第几个数据"() -> (w423:i32)
                n422 = local read "数组_设定值"() -> (w454:dbl[][])
                n423 = local read "数组_选择"() -> (w432:bool[])
                n424 = Index Array(array=w460, index #1=3 ("索引"), index #2=4 ("索引"), index #3=5 ("索引"), index #4=6 ("索引")) -> (element #1=w439:u16, element #2=w438:u16, element #3=w437:u16, element #4=w436:u16)
                n425 = local read "第几组数据"() -> (w435:i32)
                n426 = Add(x=w428, y=16) -> (x+y=w441:i32)
                n427 = call "U16转换为float.vi"("第几组数据"=w435, "选择?"=w432, "低16位_2"=w436, "高16位_2"=w437, "低16位_1"=w438, "高16位_1"=w439) -> ("反馈值2"=w430:dbl, "反馈值1"=w421:dbl, "反馈值字符_2"=w433:string, "反馈值字符_1"=w434:string)  [unwired: 2 in]
                n428 = Index Array(array=w454, index (row) #1=w428, index (col) #1=w423, index (row) #2=w441, index (col) #2=w423) -> (element #1=w422:dbl, element #2=w429:dbl)
                n429 = local read "Analog_back"() -> (w446:string[][])
                n430 = local read "第几个数据"() -> (w440:i32)
                n431 = local read "数组_选择"() -> (w431:bool[])
                n432 = Add(x=w435, y=16) -> (x+y=w444:i32)
                n433 = call "一个反馈计算误差.vi"("第几组"=w428, "选择?"=w431, "设定值_2"=w429, "设定值_1"=w422, "反馈值_2"=w430, "反馈值_1"=w421) -> ("字符串_误差_2"=w425:string, "字符串_误差_1"=w426:string, "合格_2?"=w424:bool, "合格_1?"=w427:bool)  [unwired: 2 out]
                n434 = Replace Array Subset(array=w446, new element #1=w434, index (row) #1=w435, index (col) #1=w440, new element #2=w433, index (row) #2=w444, index (col) #2=w440) -> (w445:string[][])
                n435 = local write "Analog_back"(w445) -> ()
                n436 = local read "第几个数据"() -> (w442:i32)
                n437 = local read "Analog_WC"() -> (w451:string[][])
                n438 = local read "第几组数据"() -> (w449:i32)
                n439 = Add(x=w449, y=16) -> (x+y=w443:i32)
                n440 = Replace Array Subset(array=w451, new element #1=w426, index (row) #1=w449, index (col) #1=w442, new element #2=w425, index (row) #2=w443, index (col) #2=w442) -> (w450:string[][])
                n441 = local read "合格？"() -> (w447:bool[][])
                n442 = local write "Analog_WC"(w450) -> ()
                n443 = Replace Array Subset(array=w447, new element #1=w427, index (row) #1=w449, index (col) #1=w442, new element #2=w424, index (row) #2=w443, index (col) #2=w442) -> (w448:bool[][])
                n444 = local write "合格？"(w448) -> ()
              }
              frame #1 {
                n445 = local read "合格？"() -> (w470:bool[][])
                n446 = local read "第几组数据"() -> (w464:i32)
                n447 = Add(x=w464, y=16) -> (x+y=w463:i32)
                n448 = Index Array(array=w470, index (row) #1=w464, index (row) #2=w463) -> (element #1=w473:bool[], element #2=w467:bool[])  [unwired: 2 in]
                n449 = And Array Elements(Boolean array=w473) -> (logical AND=w468:bool)
                n450 = And Array Elements(Boolean array=w467) -> (logical AND=w466:bool)
                n451 = local read "数组_选择"() -> (w465:bool[])
                n452 = Index Array(array=w465, index #1=w464, index #2=w463) -> (element #1=w462:bool, element #2=w461:bool)
                n453 = case shown="真" w462 {
                  tunnel: [cluster{u32, u32}[] [{12369084, 12369084}] w481] -> w472
                  tunnel: w468 -> [_ w480]
                  frame False {
                  }
                  frame True {
                    n454 = case shown="真" w480 {
                      tunnel: [cluster{u32, u32}[] [{16730410, 16711680}] cluster{u32, u32}[] [{61205, 6618880}]] -> w481
                      frame False {
                      }
                      frame True {
                      }
                    }
                  }
                }
                n455 = case shown="真" w461 {
                  tunnel: [cluster{u32, u32}[] [{12369084, 12369084}] w476] -> w469
                  tunnel: w466 -> [_ w475]
                  frame False {
                  }
                  frame True {
                    n456 = case shown="真" w475 {
                      tunnel: [cluster{u32, u32}[] [{16730410, 16711680}] cluster{u32, u32}[] [{61205, 6618880}]] -> w476
                      frame False {
                      }
                      frame True {
                      }
                    }
                  }
                }
                n457 = case shown="31" w464 {
                  tunnel: w472 -> [w516 w517 w518 w519 w520 w521 w522 w523 w524 w525 w526 w527 w528 w529 w530 w531 w532 w533 w534 w535 w536 w537 w538 w539 w540 w541 w542 w543 w544 w545 w546 w547]
                  frame 0, Default {
                    n458 = property on="light_1" class="Bool (严格)"("Colors [4]"=w516) -> ()  [unwired: 2 in, 2 out]
                  }
                  frame 1 {
                    n459 = property on="light_2" class="Bool (严格)"("Colors [4]"=w517) -> ()  [unwired: 2 in, 2 out]
                  }
                  frame 2 {
                    n460 = property on="light_3" class="Bool (严格)"("Colors [4]"=w518) -> ()  [unwired: 2 in, 2 out]
                  }
                  frame 3 {
                    n461 = property on="light_4" class="Bool (严格)"("Colors [4]"=w519) -> ()  [unwired: 2 in, 2 out]
                  }
                  frame 4 {
                    n462 = property on="light_5" class="Bool (严格)"("Colors [4]"=w520) -> ()  [unwired: 2 in, 2 out]
                  }
                  frame 5 {
                    n463 = property on="light_6" class="Bool (严格)"("Colors [4]"=w521) -> ()  [unwired: 2 in, 2 out]
                  }
                  frame 6 {
                    n464 = property on="light_7" class="Bool (严格)"("Colors [4]"=w522) -> ()  [unwired: 2 in, 2 out]
                  }
                  frame 7 {
                    n465 = property on="light_8" class="Bool (严格)"("Colors [4]"=w523) -> ()  [unwired: 2 in, 2 out]
                  }
                  frame 8 {
                    n466 = property on="light_9" class="Bool (严格)"("Colors [4]"=w524) -> ()  [unwired: 2 in, 2 out]
                  }
                  frame 9 {
                    n467 = property on="light_10" class="Bool (严格)"("Colors [4]"=w525) -> ()  [unwired: 2 in, 2 out]
                  }
                  frame 10 {
                    n468 = property on="light_11" class="Bool (严格)"("Colors [4]"=w526) -> ()  [unwired: 2 in, 2 out]
                  }
                  frame 11 {
                    n469 = property on="light_12" class="Bool (严格)"("Colors [4]"=w527) -> ()  [unwired: 2 in, 2 out]
                  }
                  frame 12 {
                    n470 = property on="light_13" class="Bool (严格)"("Colors [4]"=w528) -> ()  [unwired: 2 in, 2 out]
                  }
                  frame 13 {
                    n471 = property on="light_14" class="Bool (严格)"("Colors [4]"=w529) -> ()  [unwired: 2 in, 2 out]
                  }
                  frame 14 {
                    n472 = property on="light_15" class="Bool (严格)"("Colors [4]"=w530) -> ()  [unwired: 2 in, 2 out]
                  }
                  frame 15 {
                    n473 = property on="light_16" class="Bool (严格)"("Colors [4]"=w531) -> ()  [unwired: 2 in, 2 out]
                  }
                  frame 16 {
                    n474 = property on="light_17" class="Bool (严格)"("Colors [4]"=w532) -> ()  [unwired: 2 in, 2 out]
                  }
                  frame 17 {
                    n475 = property on="light_18" class="Bool (严格)"("Colors [4]"=w533) -> ()  [unwired: 2 in, 2 out]
                  }
                  frame 18 {
                    n476 = property on="light_19" class="Bool (严格)"("Colors [4]"=w534) -> ()  [unwired: 2 in, 2 out]
                  }
                  frame 19 {
                    n477 = property on="light_20" class="Bool (严格)"("Colors [4]"=w535) -> ()  [unwired: 2 in, 2 out]
                  }
                  frame 20 {
                    n478 = property on="light_21" class="Bool (严格)"("Colors [4]"=w536) -> ()  [unwired: 2 in, 2 out]
                  }
                  frame 21 {
                    n479 = property on="light_22" class="Bool (严格)"("Colors [4]"=w537) -> ()  [unwired: 2 in, 2 out]
                  }
                  frame 22 {
                    n480 = property on="light_23" class="Bool (严格)"("Colors [4]"=w538) -> ()  [unwired: 2 in, 2 out]
                  }
                  frame 23 {
                    n481 = property on="light_24" class="Bool (严格)"("Colors [4]"=w539) -> ()  [unwired: 2 in, 2 out]
                  }
                  frame 24 {
                    n482 = property on="light_25" class="Bool (严格)"("Colors [4]"=w540) -> ()  [unwired: 2 in, 2 out]
                  }
                  frame 25 {
                    n483 = property on="light_26" class="Bool (严格)"("Colors [4]"=w541) -> ()  [unwired: 2 in, 2 out]
                  }
                  frame 26 {
                    n484 = property on="light_27" class="Bool (严格)"("Colors [4]"=w542) -> ()  [unwired: 2 in, 2 out]
                  }
                  frame 27 {
                    n485 = property on="light_28" class="Bool (严格)"("Colors [4]"=w543) -> ()  [unwired: 2 in, 2 out]
                  }
                  frame 28 {
                    n486 = property on="light_29" class="Bool (严格)"("Colors [4]"=w544) -> ()  [unwired: 2 in, 2 out]
                  }
                  frame 29 {
                    n487 = property on="light_30" class="Bool (严格)"("Colors [4]"=w545) -> ()  [unwired: 2 in, 2 out]
                  }
                  frame 30 {
                    n488 = property on="light_31" class="Bool (严格)"("Colors [4]"=w546) -> ()  [unwired: 2 in, 2 out]
                  }
                  frame 31 {
                    n489 = property on="light_32" class="Bool (严格)"("Colors [4]"=w547) -> ()  [unwired: 2 in, 2 out]
                  }
                }
                n490 = case shown="31" w463 {
                  tunnel: w469 -> [w484 w485 w486 w487 w488 w489 w490 w491 w492 w493 w494 w495 w496 w497 w498 w499 w500 w501 w502 w503 w504 w505 w506 w507 w508 w509 w510 w511 w512 w513 w514 w515]
                  frame 0, Default {
                    n491 = property on="light_1" class="Bool (严格)"("Colors [4]"=w484) -> ()  [unwired: 2 in, 2 out]
                  }
                  frame 1 {
                    n492 = property on="light_2" class="Bool (严格)"("Colors [4]"=w485) -> ()  [unwired: 2 in, 2 out]
                  }
                  frame 2 {
                    n493 = property on="light_3" class="Bool (严格)"("Colors [4]"=w486) -> ()  [unwired: 2 in, 2 out]
                  }
                  frame 3 {
                    n494 = property on="light_4" class="Bool (严格)"("Colors [4]"=w487) -> ()  [unwired: 2 in, 2 out]
                  }
                  frame 4 {
                    n495 = property on="light_5" class="Bool (严格)"("Colors [4]"=w488) -> ()  [unwired: 2 in, 2 out]
                  }
                  frame 5 {
                    n496 = property on="light_6" class="Bool (严格)"("Colors [4]"=w489) -> ()  [unwired: 2 in, 2 out]
                  }
                  frame 6 {
                    n497 = property on="light_7" class="Bool (严格)"("Colors [4]"=w490) -> ()  [unwired: 2 in, 2 out]
                  }
                  frame 7 {
                    n498 = property on="light_8" class="Bool (严格)"("Colors [4]"=w491) -> ()  [unwired: 2 in, 2 out]
                  }
                  frame 8 {
                    n499 = property on="light_9" class="Bool (严格)"("Colors [4]"=w492) -> ()  [unwired: 2 in, 2 out]
                  }
                  frame 9 {
                    n500 = property on="light_10" class="Bool (严格)"("Colors [4]"=w493) -> ()  [unwired: 2 in, 2 out]
                  }
                  frame 10 {
                    n501 = property on="light_11" class="Bool (严格)"("Colors [4]"=w494) -> ()  [unwired: 2 in, 2 out]
                  }
                  frame 11 {
                    n502 = property on="light_12" class="Bool (严格)"("Colors [4]"=w495) -> ()  [unwired: 2 in, 2 out]
                  }
                  frame 12 {
                    n503 = property on="light_13" class="Bool (严格)"("Colors [4]"=w496) -> ()  [unwired: 2 in, 2 out]
                  }
                  frame 13 {
                    n504 = property on="light_14" class="Bool (严格)"("Colors [4]"=w497) -> ()  [unwired: 2 in, 2 out]
                  }
                  frame 14 {
                    n505 = property on="light_15" class="Bool (严格)"("Colors [4]"=w498) -> ()  [unwired: 2 in, 2 out]
                  }
                  frame 15 {
                    n506 = property on="light_16" class="Bool (严格)"("Colors [4]"=w499) -> ()  [unwired: 2 in, 2 out]
                  }
                  frame 16 {
                    n507 = property on="light_17" class="Bool (严格)"("Colors [4]"=w500) -> ()  [unwired: 2 in, 2 out]
                  }
                  frame 17 {
                    n508 = property on="light_18" class="Bool (严格)"("Colors [4]"=w501) -> ()  [unwired: 2 in, 2 out]
                  }
                  frame 18 {
                    n509 = property on="light_19" class="Bool (严格)"("Colors [4]"=w502) -> ()  [unwired: 2 in, 2 out]
                  }
                  frame 19 {
                    n510 = property on="light_20" class="Bool (严格)"("Colors [4]"=w503) -> ()  [unwired: 2 in, 2 out]
                  }
                  frame 20 {
                    n511 = property on="light_21" class="Bool (严格)"("Colors [4]"=w504) -> ()  [unwired: 2 in, 2 out]
                  }
                  frame 21 {
                    n512 = property on="light_22" class="Bool (严格)"("Colors [4]"=w505) -> ()  [unwired: 2 in, 2 out]
                  }
                  frame 22 {
                    n513 = property on="light_23" class="Bool (严格)"("Colors [4]"=w506) -> ()  [unwired: 2 in, 2 out]
                  }
                  frame 23 {
                    n514 = property on="light_24" class="Bool (严格)"("Colors [4]"=w507) -> ()  [unwired: 2 in, 2 out]
                  }
                  frame 24 {
                    n515 = property on="light_25" class="Bool (严格)"("Colors [4]"=w508) -> ()  [unwired: 2 in, 2 out]
                  }
                  frame 25 {
                    n516 = property on="light_26" class="Bool (严格)"("Colors [4]"=w509) -> ()  [unwired: 2 in, 2 out]
                  }
                  frame 26 {
                    n517 = property on="light_27" class="Bool (严格)"("Colors [4]"=w510) -> ()  [unwired: 2 in, 2 out]
                  }
                  frame 27 {
                    n518 = property on="light_28" class="Bool (严格)"("Colors [4]"=w511) -> ()  [unwired: 2 in, 2 out]
                  }
                  frame 28 {
                    n519 = property on="light_29" class="Bool (严格)"("Colors [4]"=w512) -> ()  [unwired: 2 in, 2 out]
                  }
                  frame 29 {
                    n520 = property on="light_30" class="Bool (严格)"("Colors [4]"=w513) -> ()  [unwired: 2 in, 2 out]
                  }
                  frame 30 {
                    n521 = property on="light_31" class="Bool (严格)"("Colors [4]"=w514) -> ()  [unwired: 2 in, 2 out]
                  }
                  frame 31 {
                    n522 = property on="light_32" class="Bool (严格)"("Colors [4]"=w515) -> ()  [unwired: 2 in, 2 out]
                  }
                }
              }
              frame #2 {
                n523 = local read "第几组数据"() -> (w551:i32)
                n524 = Add(x=w551, y=16) -> (x+y=w553:i32)
                n525 = local read "第几个数据"() -> (w555:i32)
                n526 = local read "合格？"() -> (w556:bool[][])
                n527 = local read "数组_选择"() -> (w554:bool[])
                n528 = Index Array(array=w556, index (row) #1=w551, index (col) #1=w555, index (row) #2=w553, index (col) #2=w555) -> (element #1=w552:bool, element #2=w548:bool)
                n529 = Index Array(array=w554, index #1=w551, index #2=w553) -> (element #1=w550:bool, element #2=w549:bool)
                n530 = case shown="真" w550 {
                  tunnel: w555 -> [_ w567]
                  tunnel: w552 -> [_ w566]
                  tunnel: w551 -> [_ w565]
                  frame False {
                  }
                  frame True {
                    n531 = call "误差表格颜色.vi"("合格？"=w566, "第几组"=w565) -> ("颜色"=w564:u32)  [unwired: 9 in]
                    n532 = Bundle("第几组数据"=w565, "第几个数据"=w567) -> (w569:cluster{"第几组数据":i32, "第几个数据":i32})  [unwired: 1 in]
                    n533 = property on="Analog_WC" class="Tbl (严格)"("Active Cell"=w569) -> (error out=w568:errorcluster)  [unwired: 2 in, 1 out]
                    n534 = property on="Analog_WC" class="Tbl (严格)"(error in=w568, "Cell BG Color"=w564) -> ()  [unwired: 1 in, 2 out]
                  }
                }
                n535 = case shown="真" w549 {
                  tunnel: w555 -> [_ w561]
                  tunnel: w553 -> [_ w560]
                  tunnel: w548 -> [_ w558]
                  frame False {
                  }
                  frame True {
                    n536 = Bundle(w560, "第几个数据"=w561) -> (w562:cluster{i32, "第几个数据":i32})  [unwired: 1 in]
                    n537 = call "误差表格颜色.vi"("合格？"=w558, "第几组"=w560) -> ("颜色"=w559:u32)  [unwired: 9 in]
                    n538 = property on="Analog_WC" class="Tbl (严格)"("Active Cell"=w562) -> (error out=w563:errorcluster)  [unwired: 2 in, 1 out]
                    n539 = property on="Analog_WC" class="Tbl (严格)"(error in=w563, "Cell BG Color"=w559) -> ()  [unwired: 1 in, 2 out]
                  }
                }
              }
              frame #3 {
                n540 = flat-sequence {
                  frame #0 {
                    n541 = Wait Until Next ms Multiple(millisecond multiple=u32 100) -> ()  [unwired: 1 out]
                  }
                  frame #1 {
                    n542 = local write "同步_1"(0 ("同步_1")) -> ()
                  }
                }
              }
            }
          }
        }
        n543 = case shown="真" w403 {
          frame False {
          }
          frame True {
            # "第几个"
            # "第几组"
            n544 = local read "第几个数据"() -> (w414:i32)
            n545 = local read "第几组数据"() -> (w416:i32)
            n546 = Increment(x=w416) -> (x+1=w417:i32)
            n547 = Increment(x=w414) -> (x+1=w415:i32)
            n548 = Format Into String(format string="第%d组%d个数据反馈失败（UDP）" ("Message"), w417, w415) -> (resulting string=w418:string)  [unwired: 2 in, 1 out]
            n549 = call "显示对话框信息2"("Message"=w418) -> ()  [unwired: 9 in, 2 out]
            n550 = local write "同步_1"(0 ("同步_1")) -> ()
          }
        }
      }
    }
    n551 = local read "退出？"() -> (w389:bool)
  }
  n552 = Release Notifier(notifier=w2, error in (no error)=w1) -> ()  [unwired: 1 in, 3 out]
